vi "Acquire.vi"(8 "error in (no error)":errorcluster, 10 "Msg in":T1, 11 "DG645 in":refnum<class "SMC100.lvclass">) -> (0 "error out":errorcluster, 1 "new command":string, 2 "Msg out":T1, 3 "DG645 out":refnum<class "SMC100.lvclass">)   [LabVIEW 2020, in "SMC100.lvclass"]
uses:
  SMC100.lvclass
  C:/GEECS/Developers Version/source/Device Drivers/BaseDriver/BaseDriver.lvclass
  BaseDriver/DriverMsg.ctl
  SMC100.lvclass/SMC100.ctl
  shared/CompressAndUpdate(Poly)/CompressAndUpdate(Numeric).vi
  BaseDriver/BaseDriver.lvclass
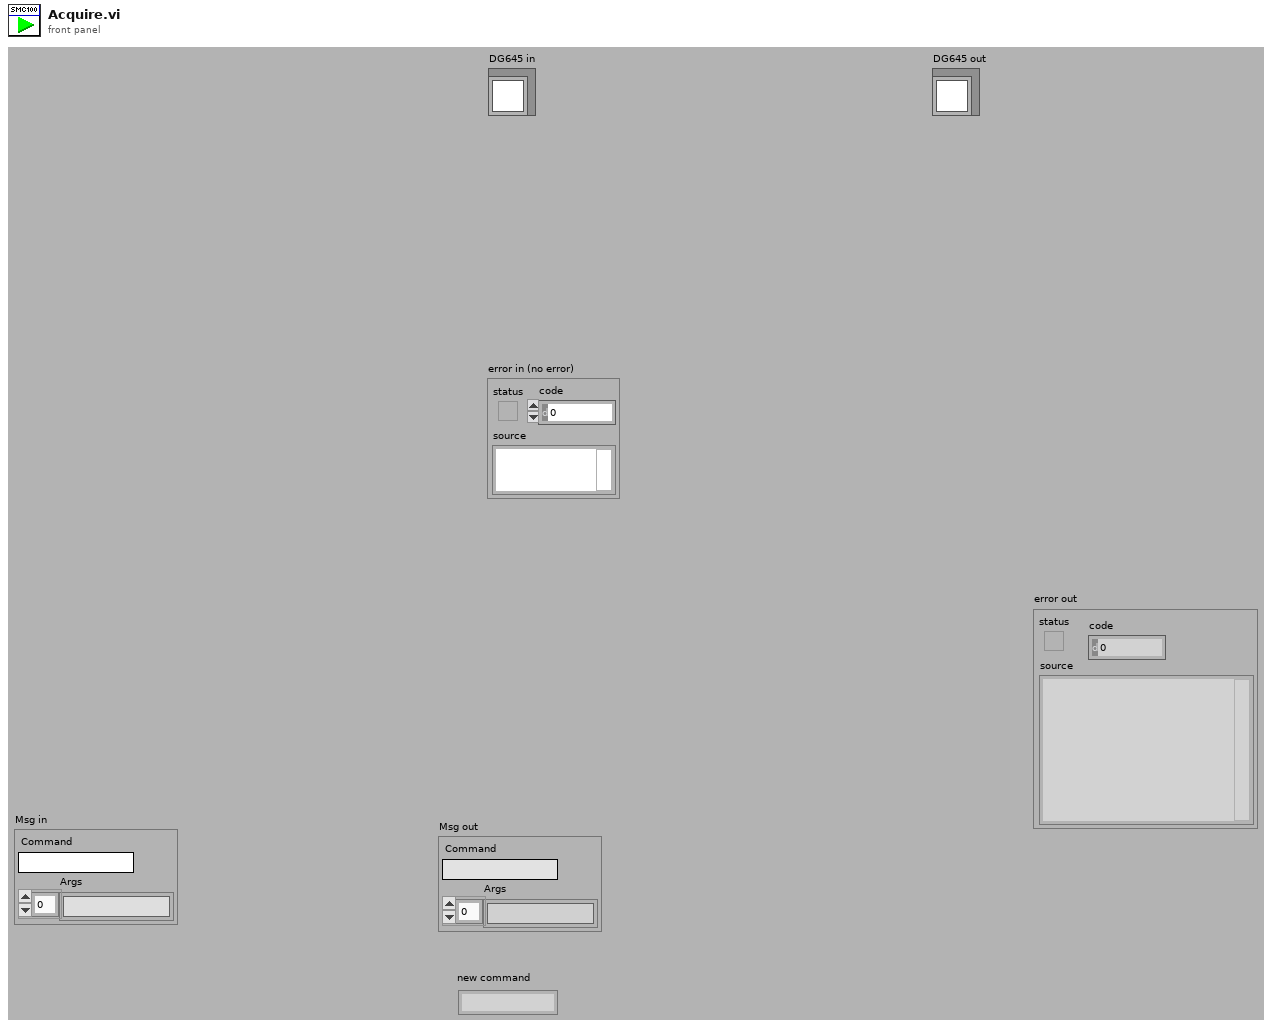
[diagram p1: front panel]
types:
  T1 = typedef "DriverMsg.ctl" = cluster{"Command":string, "Args":string[]}
  T2 = cluster{"VisaResourceName":string, "DeviceName":string, i32, "error out":errorcluster}
  T3 = cluster{"VISA resource name":refnum<visa-resource-name>, "Device name":string, "Controller address":i32, "error":errorcluster}
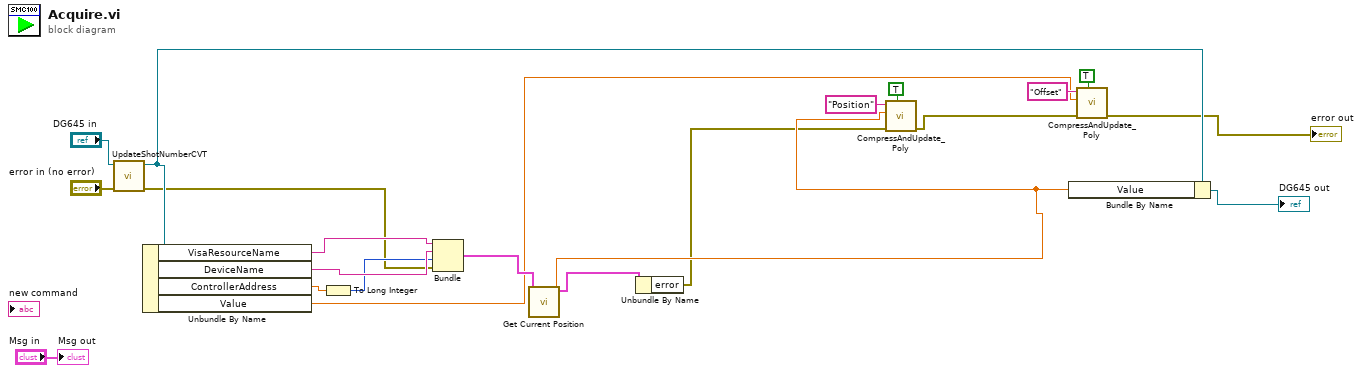
[diagram p0: block diagram]
diagram:
  n1 = call "UpdateShotNumberCVT.vi"("error in (no error)"="error in (no error)", "BaseDriver in"="DG645 in") -> ("error out"=w10:errorcluster, "BaseDriver out"=w15:refnum<class "SMC100.lvclass">)  [unwired: 8 in]
  n2 = Unbundle By Name(w15) -> ("VisaResourceName"=w13:string, "DeviceName"=w12:string, "ControllerAddress"=w14:dbl, "Value"=w1:dbl)
  n3 = To Long Integer(number=w14) -> (32bit integer=w11:i32)
  n4 = Bundle("VisaResourceName"=w13, "DeviceName"=w12, w11, "error out"=w10) -> (w9:T2)  [unwired: 1 in]
  n5 = call "Get Current Position.vi"("Connection Cluster in"=w9) -> ("Current position"=w7:dbl, "Connection Cluster out"=w8:T3)  [unwired: 8 in, 1 out]
  n6 = Unbundle By Name(w8) -> ("error"=w4:errorcluster)
  n7 = call-poly "CompressAndUpdate_Poly.vi"("force CVT update (false)"=TRUE, "error in"=w4, "Numeric"=w7, "command or variable name"="Position") -> ("error out"=w3:errorcluster)  [unwired: 7 in]
  n8 = Bundle By Name(cluster=w15, "Value"=w7) -> (→"DG645 out":refnum<class "SMC100.lvclass">)
  n9 = call-poly "CompressAndUpdate_Poly.vi"("force CVT update (false)"=TRUE, "error in"=w3, "Numeric"=w1, "command or variable name"="Offset") -> ("error out"=→"error out":errorcluster)  [unwired: 7 in]
  "Msg out" <- "Msg in"
